vi "CenterFinder_6points.vi"() -> ()   [LabVIEW 2016]
uses:
  Control/ProcessCtl.ctl
  <vilib>/userdefined/High Color/IMAQdx.ctl
  <vilib>/Utility/config.llb/Read Key (String).vi
  <vilib>/Utility/config.llb/Write Key (Double).vi
  <vilib>/vision/driver/NI_Vision_Acquisition_Software.lvlib
  <vilib>/vision/NI_Vision_Development_Module.lvlib
  <vilib>/Utility/config.llb/NI_LVConfig.lvlib
panel:
  out "Array":T1(array[cluster])
  in  "MoveTo":bool
  out "Boolean":bool=TRUE
  in  "GoToXY":bool
  out "Tip Center":cluster{"X":dbl, "Y":dbl, "Z":dbl}
  in  "Minimum Edge Strength":dbl=10.0
  out "Camera Center":cluster{"X":dbl, "Y":dbl, "Z":dbl}
  out "1":bool[](array[boolean])
  in  "LR/TB":enum16{"B2T", "L2R", "R2L", "T2B"}(ring)=enum."R2L"
  in  "Delete":bool caption="Retake"
  in  "Retake":bool caption="Delete"
  in  "Next":bool
  in  "Process":bool
  in  "Acquire":bool
  in  "stop":bool
  out "Image":T2(plugin-control)
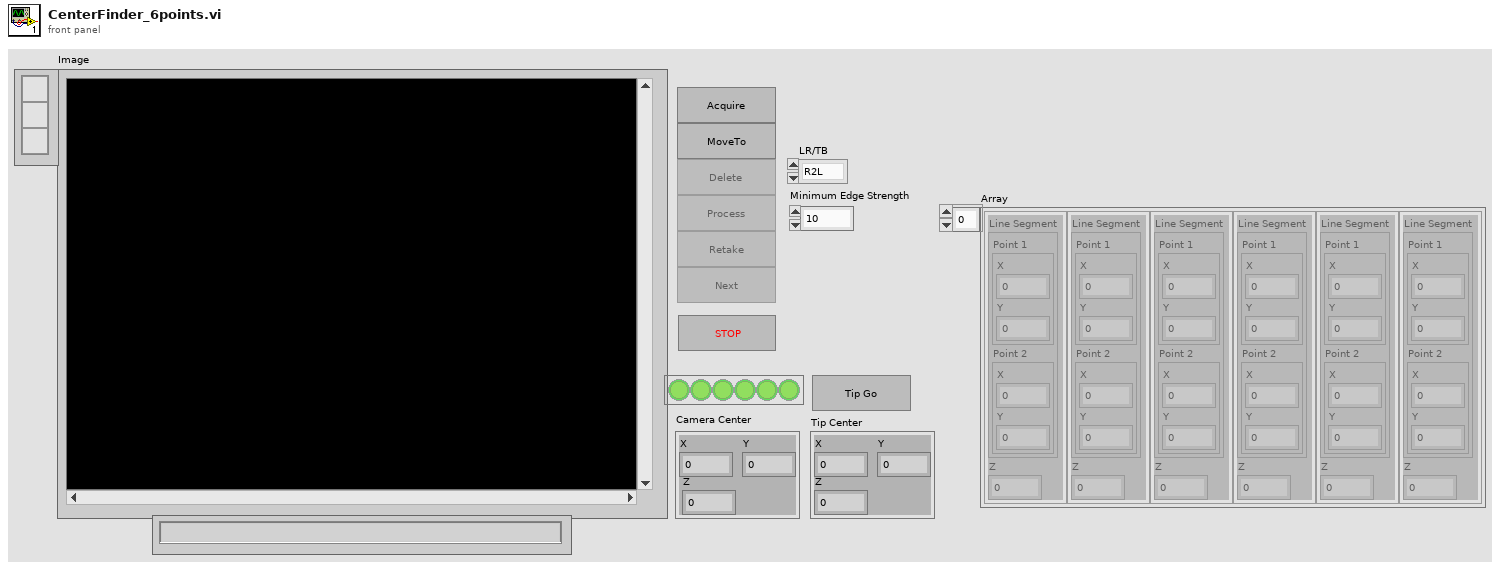
[diagram p1: front panel]
types:
  T1 = cluster{"Line Segment":cluster{"Point 1":cluster{"X":sgl, "Y":sgl}, "Point 2":cluster{"X":sgl, "Y":sgl}}, "Z":dbl}[]
  T2 = typedef "IMAQ Image.ctl" = refnum<image>
  T3 = typedef "IMAQdx.ctl" = refnum<k21>
  T4 = typedef "ProcessCtl.ctl" = enum16{"Idle", "Acquire", "Process", "Abort", "Initialize", "Wait"}
  T5 = typedef "NI_LVConfig.lvlib/Config Data RefNum.ctl" = refnum<k1>
  T6 = enum8{"Enabled", "Disabled", "Disabled and Grayed Out"}
  T7 = cluster{"Line Segment":cluster{"Point 1":cluster{"X":sgl, "Y":sgl}, "Point 2":cluster{"X":sgl, "Y":sgl}}, "Z":dbl}
  T8 = cluster{"Edge Polarity":u16, "Kernel Size":u32, "Width":u32, "Minimum Edge Strength":dbl, "Interpolation Type":u16, "Data Processing Method":u16}
  T9 = typedef "Image Type" = u32
  T10 = typedef "IMAQ Line" = cluster{"Start X":i32, "Start Y":i32, "End X":i32, "End Y":i32}
  T11 = typedef "ROI Descriptor" = cluster{"Global Rectangle":i32[], "Contours":cluster{"ID":enum32{"External", "Internal"}, "Type":u32, "Coordinates":i32[]}[]}
  T12 = typedef "Edge New.ctl" = cluster{"Location (Pixel)":cluster{"X":sgl, "Y":sgl}, "Location (Real-World)":cluster{"X":sgl, "Y":sgl}, "Distance (Pixel)":dbl, "Distance (Real-World)":dbl, "Strength":dbl, "Noise":dbl, "Rising?":bool}
  T13 = cluster{"Point 1":cluster{"X":sgl, "Y":sgl}, "Point 2":cluster{"X":sgl, "Y":sgl}}
  T14 = typedef "ControllerDiagPacket.ctl" = cluster{"Number of Diag Packets":i32, "Axes":T15[], "error":errorcluster}
  T15 = typedef "AxisDiagPacket.ctl" = cluster{"Axis Name":string, "Analog Input 0":dbl, "Analog Input 1":dbl, "Axis Fault (num)":i32, "Axis Fault (str)":string, "Axis Fault (bits)":cluster{"AmplifierFault":bool, "AmplifierTemperatureFault":bool, "CcwEndOfTravelLimitFault":bool, "CcwSoftwareLimitFault":bool, "CommunicationLostFault":bool, "CwEndOfTravelLimitFault":bool, "CwSoftwareLimitFault":bool, "EmergencyStopFault":bool, "EncoderFault":bool, "ExternalFault":bool, "FeedbackScalingFault":bool, "GantryMisalignFault ":bool, "HallSensorFault":bool, "InPositionTimeoutFault":bool, "InternalFault":bool, "MarkerSearchFault":bool, "MaxVelocityCommandFault":bool, "MissedInterruptFault":bool, "MotorTemperatureFault":bool, "None":bool, "OverCurrentFault":bool, "PositionErrorFault":bool, "PositionFeedbackFault":bool, "PowerSupplyFault":bool, "ProbeInputFault":bool, "SafeZoneFault":bool, "VelocityErrorFault":bool, "VelocityFeedbackFault":bool, "VoltageClampFault":bool}, "Axis Status (num)":i32, "Axis Status (str)":string, "Axis Status (bits)":cluster{"BacklashActive":bool, "CalibrationEnabled1D":bool, "CalibrationEnabled2D":bool, "CommandValid":bool, "DriveAbortPending":bool, "DrivePending":bool, "Enabling":bool, "GainMappingEnabled":bool, "GantryAligned":bool, "GantryRealigning":bool, "Homed":bool, "Homing":bool, "IFOVEnabled":bool, "JogGenerating":bool, "Jogging":bool, "JoystickControl":bool, "MasterSlaveControl":bool, "MotionBlocked":bool, "MotionClamped":bool, "MoveDone":bool, "None":bool, "NotVirtual":bool, "Profiling":bool, "Stability0":bool, "Stability1":bool, "TrajectoryFiltering":bool, "WaitDone":bool}, "Current Command":sgl, "Current Error":sgl, "Current Feedback":sgl, "Digital Inputs":i32, "Digital Outputs":i32, "Drive Status":i32, "Drive Status (str)":string, "Drive Status (bits)":cluster{"AccelerationPhase":bool, "AutofocusActive":bool, "BrakeOutput":bool, "CcwEndOfTravelLimitInput":bool, "CosineEncoderError":bool, "CurrentClamp":bool, "CwEndOfTravelLimitInput":bool, "DecelerationPhase":bool, "DualLoopActive":bool, "EmergencyStopInput":bool, "Enabled":bool, "EncoderClipping":bool, "GalvoCalibrationEnabled":bool, "GalvoPowerCorrection":bool, "HallAInput":bool, "HallBInput":bool, "HallCInput":bool, "HighResolutionMode":bool, "HomeLimitInput":bool, "InPosition":bool, "InPosition2":bool, "MarkerInput":bool, "MarkerLatch":bool, "MoveActive":bool, "NoMotorSupply":bool, "None":bool, "PowerLimiting":bool, "ProgrammingFlash":bool, "ProgrammingMXH":bool, "PSOHaltLatch":bool, "ServoControl":bool, "SineEncoderError":bool}, "Position Feedback Auxiliary":dbl, "Position Command":dbl, "Position Error":dbl, "Position Feedback":dbl, "Program Position Command":dbl, "Program Position Error":dbl, "Program Position Feedback":dbl, "Velocity Command":dbl, "Velocity Error":dbl, "Velocity Feedback":dbl}
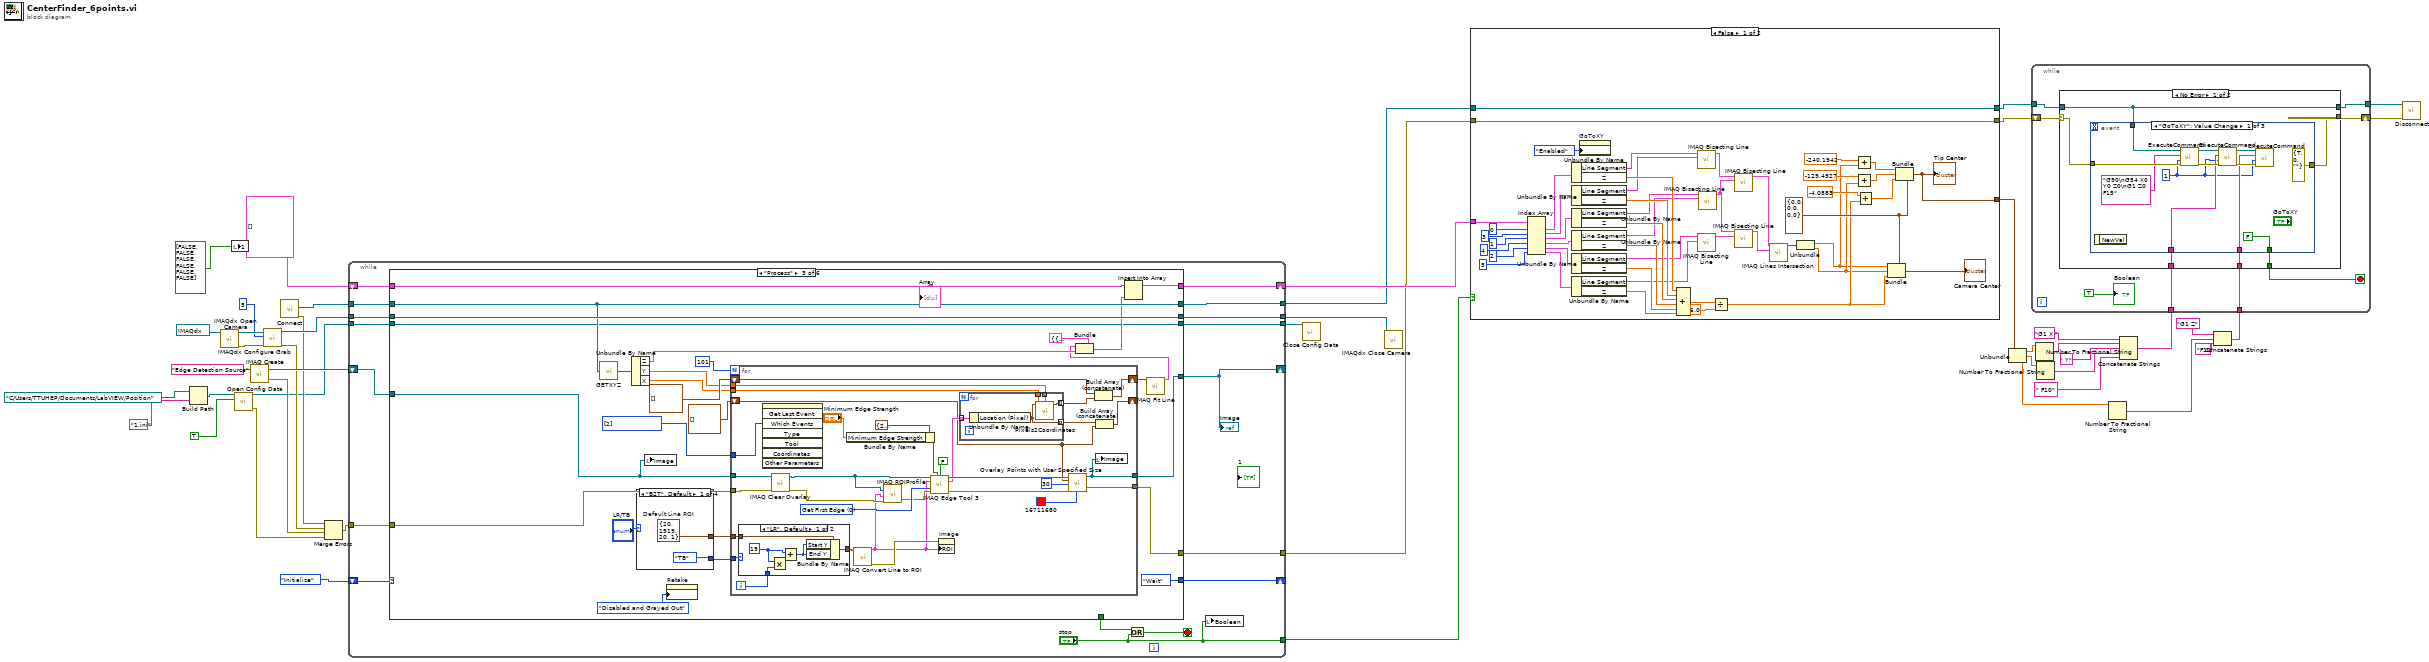
[diagram p0: block diagram]
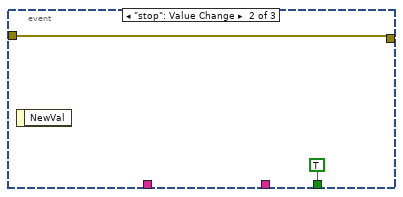
[diagram p2: hidden frame]
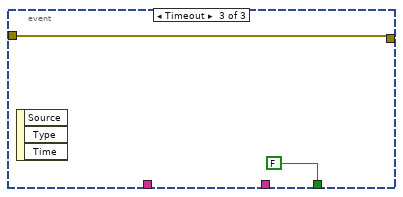
[diagram p3: hidden frame]
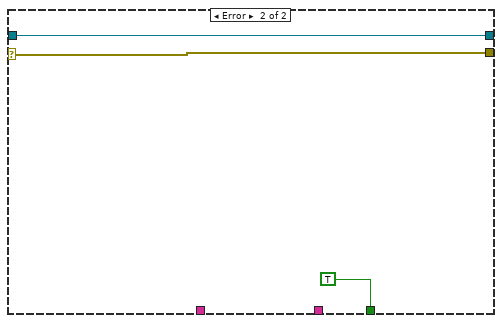
[diagram p4: hidden frame]
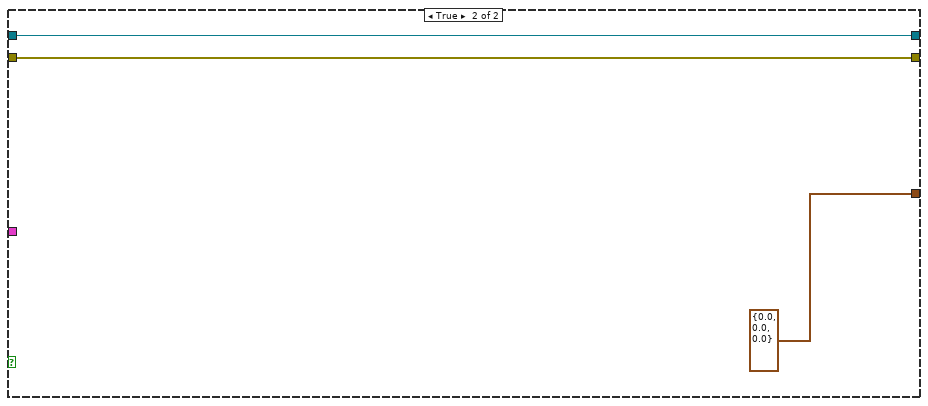
[diagram p5: hidden frame]
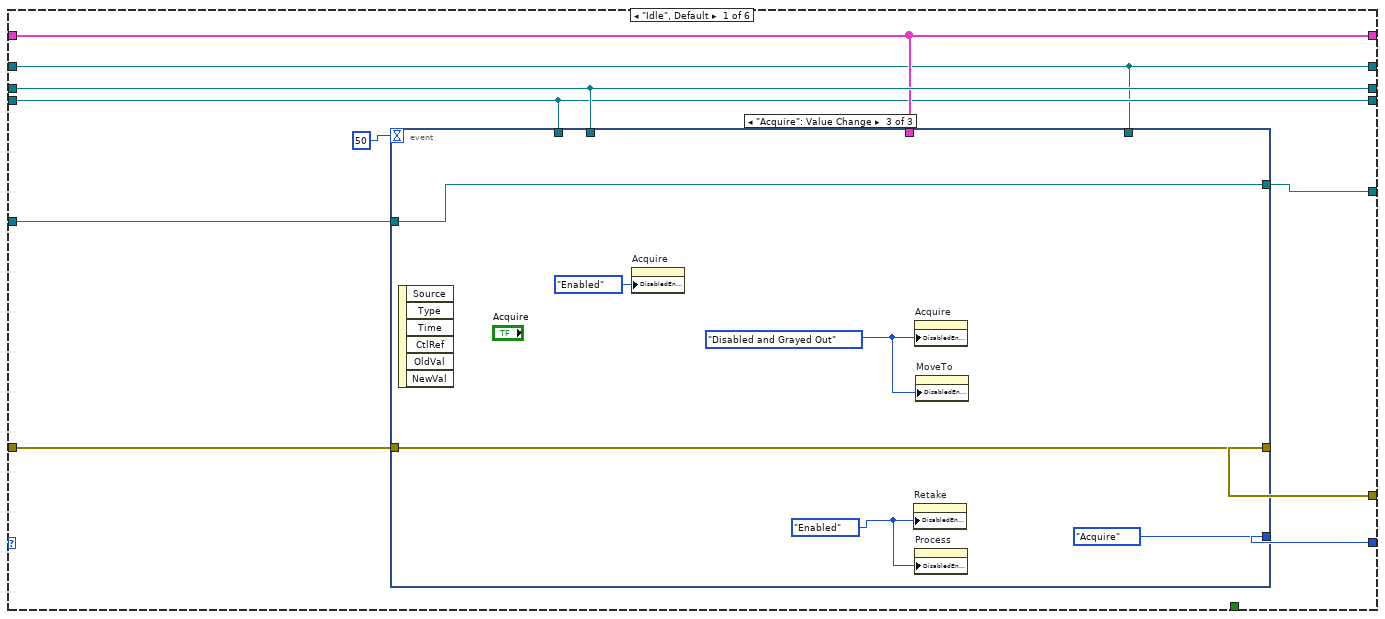
[diagram p6: hidden frame]
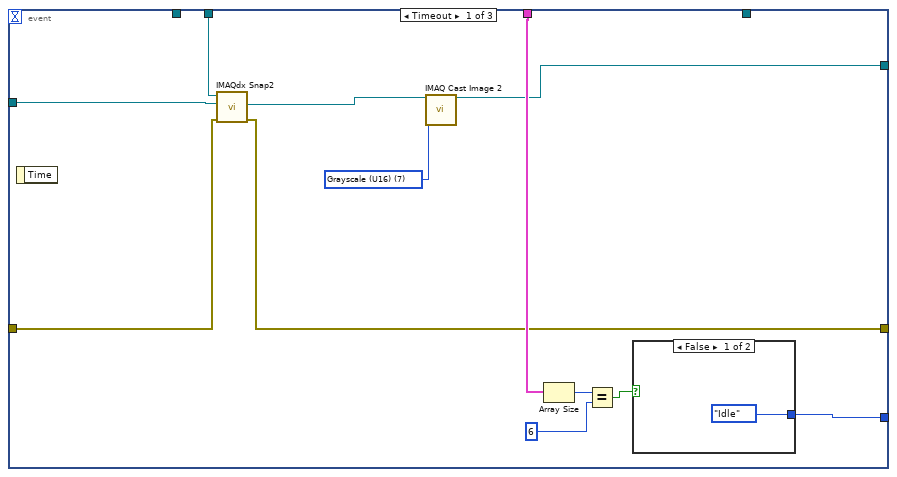
[diagram p7: hidden frame]
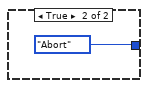
[diagram p8: hidden frame]
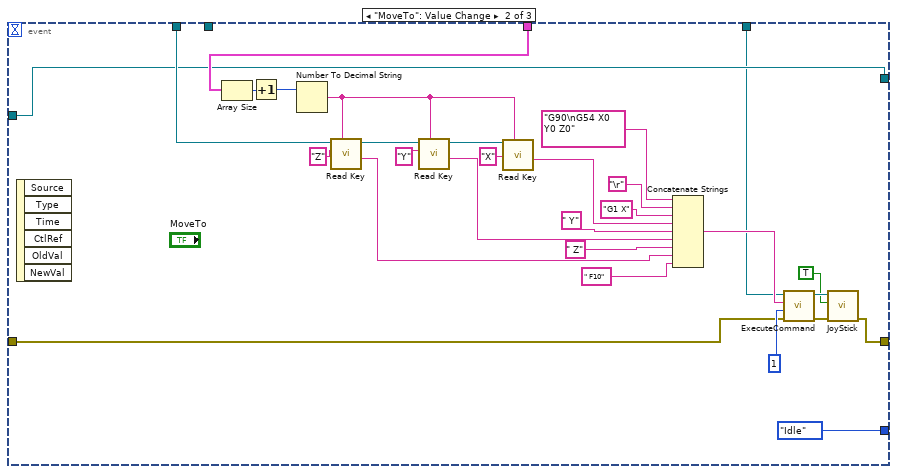
[diagram p9: hidden frame]
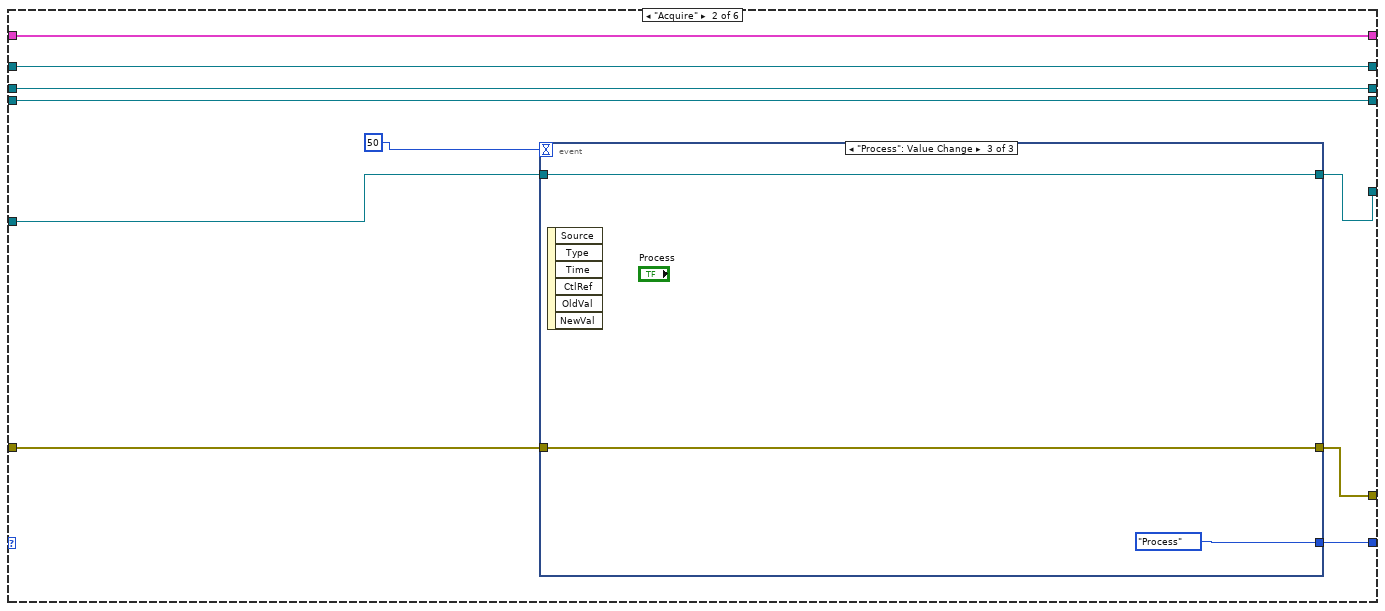
[diagram p10: hidden frame]
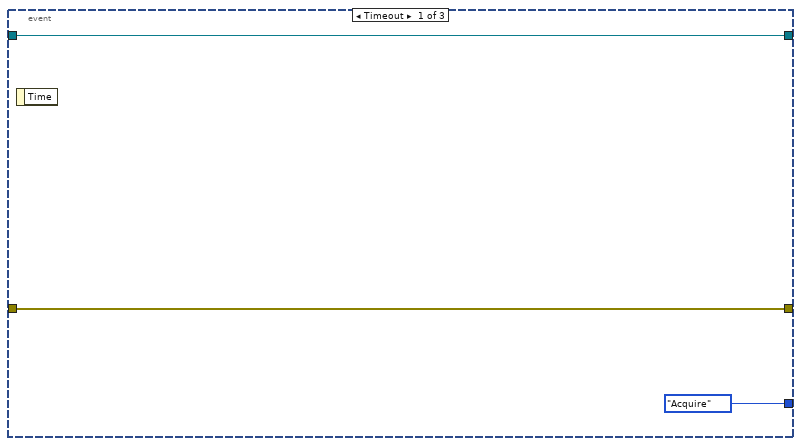
[diagram p11: hidden frame]
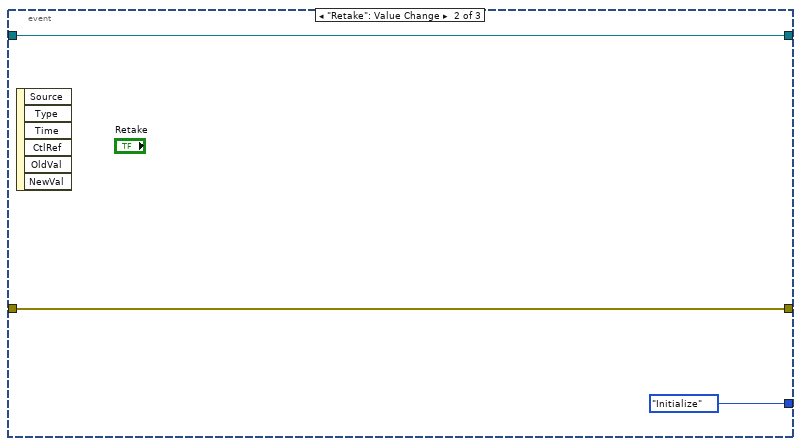
[diagram p12: hidden frame]
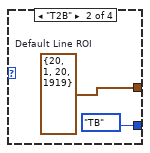
[diagram p13: hidden frame]
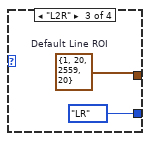
[diagram p14: hidden frame]
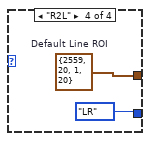
[diagram p15: hidden frame]
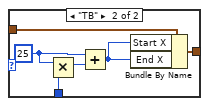
[diagram p16: hidden frame]
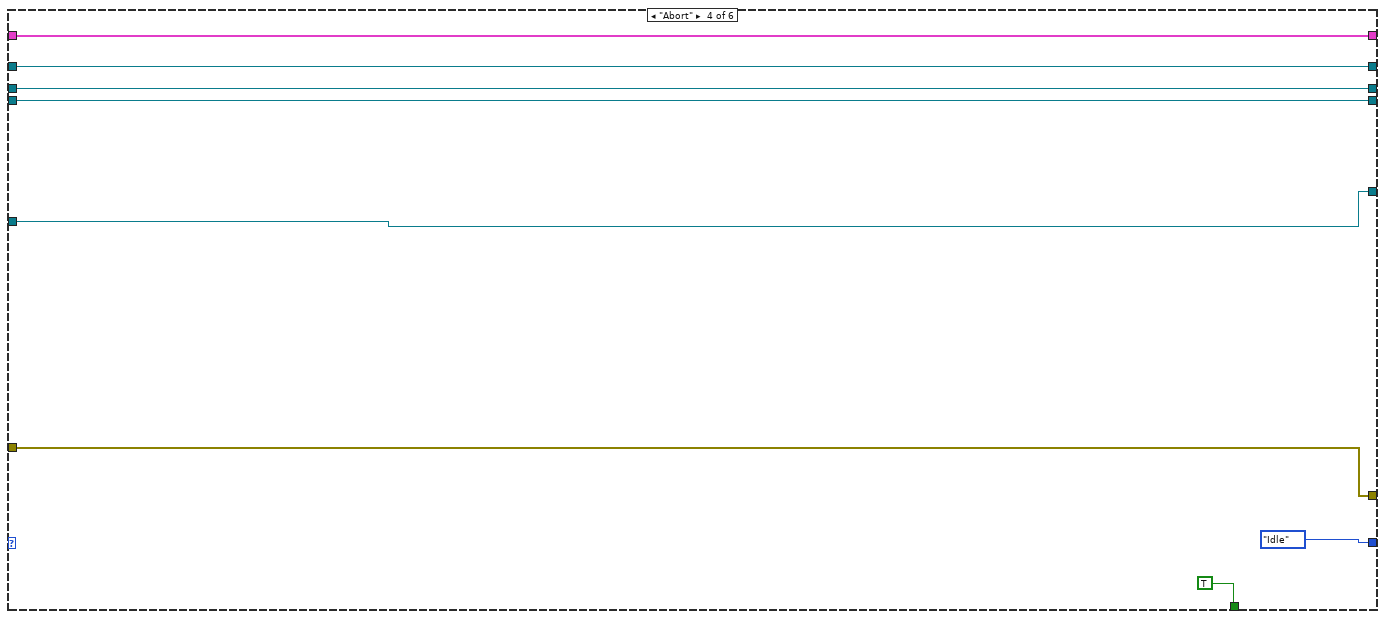
[diagram p17: hidden frame]
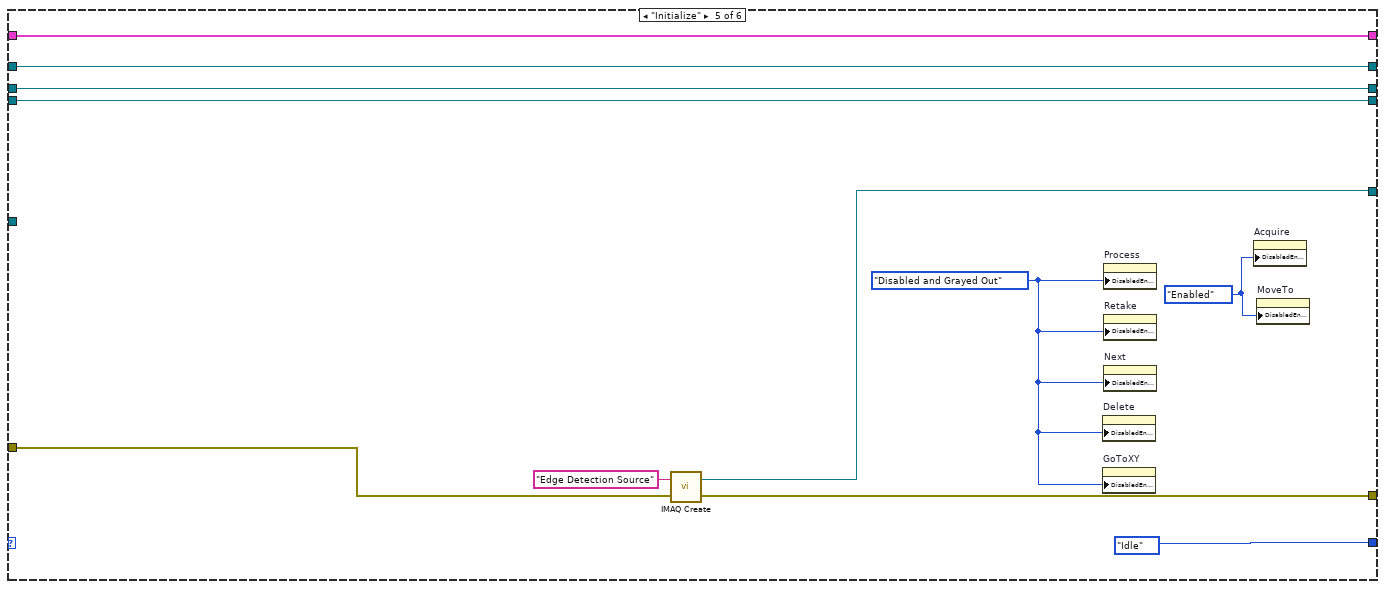
[diagram p18: hidden frame]
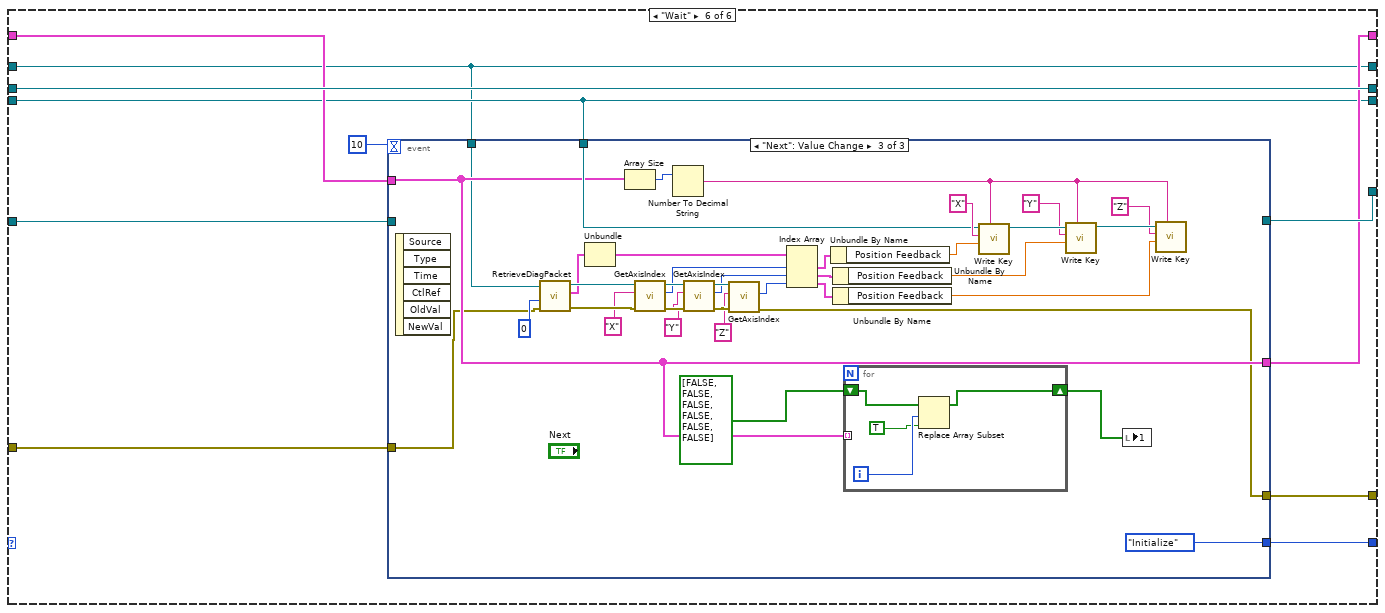
[diagram p19: hidden frame]
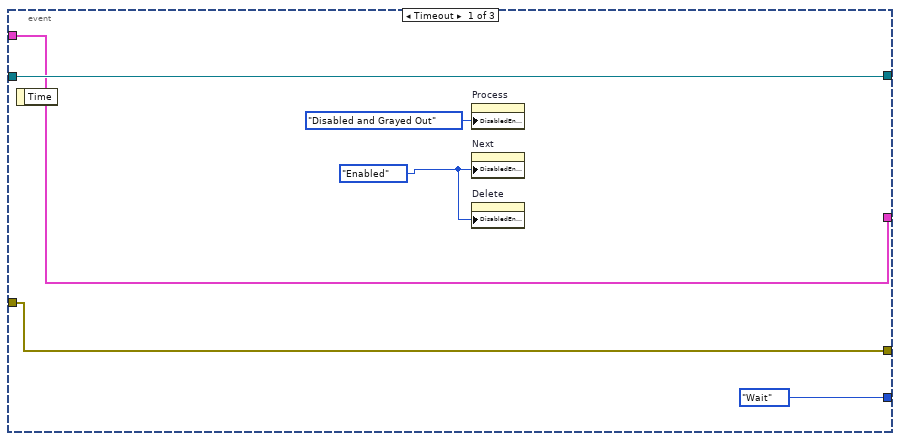
[diagram p20: hidden frame]
diagram:
  n1 = Build Path(base path=path "C:/Users/TTUHEP/Documents/LabVIEW/Position", name or relative path="1.ini") -> (appended path=w6:path)
  n2 = call <vilib>:"IMAQdx Open Camera.vi"("Session In"=T3 "cam0") -> ("error out"=w42:errorcluster, "Session Out"=w43:T3)  [unwired: 9 in]
  n3 = local write "1"(bool[] [FALSE, FALSE, FALSE, FALSE, FALSE, FALSE] ("1 2")) -> ()
  n4 = call <vilib>:"Open Config Data.vi"("create file if necessary (T)"=TRUE, "configuration file path"=w6) -> ("error out"=w5:errorcluster, "refnum"=w4:T5)  [unwired: 7 in, 1 out]
  n5 = call "IMAQ Create"("Image Name"="Edge Detection Source") -> ("New Image"=w40:T2, "error out"=w36:errorcluster)  [unwired: 4 in]
  n6 = call <vilib>:"IMAQdx Configure Grab.vi"("error in"=w42, "Number of Buffers"=u32 5, "Session In"=w43) -> ("error out"=w37:errorcluster, "Session Out"=w44:T3)  [unwired: 7 in]
  n7 = call "Connect.vi"() -> ("error out"=w15:errorcluster, "controller"=w16:refnum<k24>)  [unwired: 10 in]
  n8 = Merge Errors(w15, w37, w36, w5) -> (w35:errorcluster)
  n9 = while {
    tunnel: w44 -> [w53]
    tunnel: [w52] -> w38
    shift-right: [w59] -> _
    shift-left: w40 -> [w57]
    tunnel: w16 -> [w55]
    tunnel: [w54] -> w28
    tunnel: w35 -> [w62]
    shift-right: [w60] -> _
    shift-left: ProcessCtl."Initialize" -> [w61]
    tunnel: [w58] -> w29
    shift-right: [w49] -> w31
    shift-left: T1 [] -> [w56]
    tunnel: ["stop"] -> w30
    tunnel: w4 -> [w47]
    tunnel: [w46] -> w3
    stop <- w50 stop-if-true
    n10 = case shown="\"Process\"" w61 {
      tunnel: w62 -> [w72 w127 w165 w226 w239 w246]
      tunnel: [w69 w128 ProcessCtl."Wait" ProcessCtl."Idle" ProcessCtl."Idle" w251] -> w60
      tunnel: w57 -> [w71 w131 w147 w229 _ w253]
      tunnel: [w70 w130 w157 w229 w240 w252] -> w59
      tunnel: [w68 w126 w151 w226 w238 w247] -> w58
      tunnel: w56 -> [w66 w125 w153 w231 w237 w249]
      tunnel: [w66 w125 w152 w231 w237 w248] -> w49
      tunnel: w55 -> [w64 w124 w154 w225 w236 w243]
      tunnel: [w64 w124 w154 w225 w236 w243] -> w54
      tunnel: w53 -> [w67 w123 w155 w230 w235 w250]
      tunnel: [w67 w123 w155 w230 w235 w250] -> w52
      tunnel: [_ _ _ TRUE _ _] -> w51
      tunnel: [w65 w122 w141 w224 w233 w244] -> w46
      tunnel: w47 -> [w65 w122 w141 w224 w233 w244]
      frame "Idle", Default {
        n11 = event shown="[2] \"Acquire\": Value Change" {
          selector: _ -> [_ _ _]
          dyn-events: _ -> [_ _ _]
          timeout: 50 -> [_ _ _]
          tunnel: w72 -> [w75 w88 w118]
          tunnel: w71 -> [w77 w93 w120]
          tunnel: w67 -> [w76 _ _]
          tunnel: [w78 w93 w120] -> w70
          tunnel: [w84 ProcessCtl."Idle" ProcessCtl."Acquire"] -> w69
          tunnel: [w74 w90 w118] -> w68
          tunnel: w66 -> [w83 w114 _]
          tunnel: w65 -> [_ w115 _]
          tunnel: w64 -> [_ w87 _]
          event Timeout {
            w79 = T9 7 items=["Grayscale (U8)", "Grayscale (I16)", "Grayscale (SGL)", "Complex (CSG)", "RGB (U32)", "HSL (U32)", "RGB (U64)", "Grayscale (U16)"] ("Image Type")
            n12 = event-data() -> ()  [unwired: 1 in, 1 out]
            n13 = call <vilib>:"IMAQdx Snap2.vi"("error in"=w75, "Image In"=w77, "Session In"=w76) -> ("error out"=w74:errorcluster, "Image Out"=w73:T2)  [unwired: 6 in, 1 out]
            n14 = call "IMAQ Cast Image 2"("Image Src"=w73, "Image Type"=w79) -> ("Image Dst Out"=w78:T2)  [unwired: 12 in, 1 out]
            n15 = Array Size(array=w83) -> (size(s)=w82:i32)
            n16 = Equal?(x=w82, y=6) -> (x = y?=w80:bool)
            n17 = case shown="False" w80 {
              tunnel: [ProcessCtl."Idle" ProcessCtl."Abort"] -> w84
              frame False {
              }
              frame True {
              }
            }
          }
          event "MoveTo": Value Change {
            n18 = event-data() -> ()  [unwired: 1 in, 6 out]
            n19 = Array Size(array=w114) -> (size(s)=w113:i32)
            n20 = Increment(x=w113) -> (x+1=w95:i32)
            n21 = Number To Decimal String(number=w95) -> (decimal integer string=w112:string)  [unwired: 1 in]
            n22 = call-poly <vilib>:"Read Key.vi"("section"=w112, "key"="Z", "refnum"=w115) -> ("value"=w101:string, "refnum out"=w108:T5)  [unwired: 5 in, 2 out]
            n23 = call-poly <vilib>:"Read Key.vi"("section"=w112, "key"="Y", "refnum"=w108) -> ("value"=w102:string, "refnum out"=w107:T5)  [unwired: 5 in, 2 out]
            n24 = call-poly <vilib>:"Read Key.vi"("section"=w112, "key"="X", "refnum"=w107) -> ("value"=w103:string)  [unwired: 5 in, 3 out]
            n25 = Concatenate Strings("G90\nG54 X0 Y0 Z0", "\r", "G1 X", w103, " Y", w102, " Z", w101, " F10") -> (w97:string)
            n26 = call "ExecuteCommand.vi"("error in (no error)"=w88, "taskId"=1, "Command Code"=w97, "controller in"=w87) -> ("error out"=w91:errorcluster, "controller out"=w92:refnum<k24>)  [unwired: 5 in, 1 out]
            n27 = call "JoyStick.vi"("error in (no error)"=w91, "On/Off"=TRUE, ".NET Refnum in"=w92) -> ("error out"=w90:errorcluster)  [unwired: 7 in, 1 out]
          }
          event "Acquire": Value Change {
            w119 = T6."Enabled" ("Disabled")
            w117 = T6."Disabled and Grayed Out" ("Disabled")
            n28 = event-data() -> ()  [unwired: 1 in, 6 out]
            n29 = property on="Acquire" class="Bool"("DisabledEnum"=T6."Enabled" ("Disabled")) -> ()  [unwired: 2 in, 2 out]
            n30 = property on="Retake" class="Bool"("DisabledEnum"=w119) -> ()  [unwired: 2 in, 2 out]
            n31 = property on="Acquire" class="Bool"("DisabledEnum"=w117) -> ()  [unwired: 2 in, 2 out]
            n32 = property on="Process" class="Bool"("DisabledEnum"=w119) -> ()  [unwired: 2 in, 2 out]
            n33 = property on="MoveTo" class="Bool"("DisabledEnum"=w117) -> ()  [unwired: 2 in, 2 out]
          }
        }
      }
      frame "Acquire" {
        n34 = event shown="[2] \"Process\": Value Change" {
          selector: _ -> [_ _ _]
          dyn-events: _ -> [_ _ _]
          timeout: 50 -> [_ _ _]
          tunnel: w131 -> [w134 w135 w138]
          tunnel: [w134 w135 w138] -> w130
          tunnel: [ProcessCtl."Acquire" ProcessCtl."Initialize" ProcessCtl."Process"] -> w128
          tunnel: w127 -> [w132 w136 w139]
          tunnel: [w132 w136 w139] -> w126
          event Timeout {
            n35 = event-data() -> ()  [unwired: 1 in, 1 out]
          }
          event "Retake": Value Change {
            n36 = event-data() -> ()  [unwired: 1 in, 6 out]
          }
          event "Process": Value Change {
            n37 = event-data() -> ()  [unwired: 1 in, 6 out]
          }
        }
      }
      frame "Process" {
        w166 = i32[] [2] items=["No  event", "Click event", "Draw event", "Move event", "Size event", "Scroll event", "Activate event", "Close event", "Double click event"] ("Events list (all)")
        n38 = call "GETXYZ.vi"(".NET Refnum in"=w154) -> ("XYZ"=w160:cluster{"X":dbl, "Y":dbl, "Z":dbl})
        n39 = Unbundle By Name(w160) -> ("Z"=w144:dbl, "Y"=w159:dbl, "X"=w158:dbl)
        n40 = case shown="\"B2T\", Default" "LR/TB" {
          tunnel: [w168 w170 w171 w173] -> w163
          tunnel: [enum16{"LR", "TB"}."TB" enum16{"LR", "TB"}."TB" enum16{"LR", "TB"}."LR" enum16{"LR", "TB"}."LR"] -> w148
          frame "B2T", Default {
            w168 = T10 {"Start X"=20, "Start Y"=1919, "End X"=20, "End Y"=1}  # Default Line ROI
          }
          frame "T2B" {
            w170 = T10 {"Start X"=20, "Start Y"=1, "End X"=20, "End Y"=1919}  # Default Line ROI
          }
          frame "L2R" {
            w171 = T10 {"Start X"=1, "Start Y"=20, "End X"=2559, "End Y"=20}  # Default Line ROI
          }
          frame "R2L" {
            w173 = T10 {"Start X"=2559, "Start Y"=20, "End X"=1, "End Y"=20}  # Default Line ROI
          }
        }
        n41 = local write "Image"(w147) -> ()
        n42 = property on="Retake" class="Bool"("DisabledEnum"=T6."Disabled and Grayed Out" ("Disabled")) -> ()  [unwired: 2 in, 2 out]
        n43 = for {
          N: 101 -> [_]
          tunnel: w147 -> [w186]
          tunnel: w165 -> [w204]
          shift-right: [w196] -> w161
          shift-left: cluster{"X":sgl, "Y":sgl}[] [] -> [w198]
          tunnel: w166 -> [w190]
          tunnel: [w181] -> w157
          tunnel: [w195] -> w151
          tunnel: w163 -> [w193]
          tunnel: w159 -> [w192]
          tunnel: w158 -> [w191]
          tunnel: w148 -> [w188]
          shift-right: [w180] -> _
          shift-left: cluster{"X":sgl, "Y":sgl}[] [] -> [w178]
          i -> [w206]
          w203 = u16 0 items=["Get First Edge", "Get First + Last Edge", "Get All Edges", "Get Best Edge"] ("Process")
          n44 = case shown="\"LR\", Default" w188 {
            tunnel: w206 -> [w210 w218]
            tunnel: [w212 w214] -> w205
            tunnel: w193 -> [w211 w213]
            frame "LR", Default {
              w207 = 19
              n45 = Multiply(x=w207, y=w210) -> (x*y=w208:i32)
              n46 = Add(x=w207, y=w208) -> (x+y=w209:i32)
              n47 = Bundle By Name(cluster=w211, "Start Y"=w209, "End Y"=w209) -> (w212:T10)
            }
            frame "TB" {
              w216 = 25
              n48 = Multiply(x=w216, y=w218) -> (x*y=w217:i32)
              n49 = Add(x=w216, y=w217) -> (x+y=w215:i32)
              n50 = Bundle By Name(cluster=w213, "Start X"=w215, "End X"=w215) -> (w214:T10)
            }
          }
          n51 = invoke on="Image" class="ImageControl" method="Get Last Event"("Which Events"=w190) -> ()  [unwired: 7 in, 8 out]
          n52 = call "IMAQ Clear Overlay"("error in (no error)"=w204, "Image"=w186) -> ("error out"=w184:errorcluster, "Image Out"=w182:T2)  [unwired: 8 in]
          n53 = Bundle By Name(cluster=T8 {"Edge Polarity"=2, "Kernel Size"=37, "Width"=5, "Minimum Edge Strength"=10.0, "Interpolation Type"=0, "Data Processing Method"=1} ("Edge Options"), "Minimum Edge Strength"="Minimum Edge Strength") -> (w176:T8)
          n54 = call "IMAQ Convert Line to ROI"("Line"=w205) -> ("error out"=w189:errorcluster, "ROI Descriptor"=w183:T11)  [unwired: 8 in]
          n55 = call "IMAQ ROIProfile"("error in (no error)"=w184, "ROI Descriptor"=w183, "Image"=w182) -> ("error out"=w185:errorcluster)  [unwired: 1 in, 4 out]
          n56 = call "IMAQ Edge Tool 3"("Image"=w182, "Edge Options"=w176, "Optimized Mode"=FALSE, "ROI Descriptor"=w183, "Process"=w203, "error in (no error)"=w185) -> ("Image (duplicate)"=w201:T2, "Edge Information"=w187:T12[], "error out"=w200:errorcluster)  [unwired: 5 in, 2 out]
          n57 = property on="Image" class="ImageControl"(error in=w189, "ROI"=w183) -> ()  [unwired: 1 in, 2 out]
          n58 = for {
            tunnel: w187 -> [w223] mode=indexing
            tunnel: [w222] -> w197 mode=indexing
            tunnel: w192 -> [w221]
            tunnel: w191 -> [w220]
            tunnel: [w219] -> w179 mode=indexing
            n59 = Unbundle By Name(w223) -> ("Location (Pixel)"=w219:cluster{"X":sgl, "Y":sgl})
            n60 = call "Pixels2Coordinates.vi"("Y"=w221, "X"=w220, "Location (Pixel)"=w219) -> ("output cluster"=w222:cluster{"X":sgl, "Y":sgl})  [unwired: 8 in]
          }
          n61 = call "Overlay Points with User Specified Size.vi"("Color"=u32 16711680, "error in"=w200, "Point Diameter (5)"=30, "Points"=w178, "Image In"=w201) -> ("error out"=w195:errorcluster, "Image Out"=w181:T2)  [unwired: 5 in]
          n62 = Build Array (concatenate)(w198, w197) -> (w196:cluster{"X":sgl, "Y":sgl}[])
          n63 = Build Array (concatenate)(w179, w178) -> (w180:cluster{"X":sgl, "Y":sgl}[])
          n64 = local write "Image"(w181) -> ()
        }
        n65 = call "IMAQ Fit Line"("Points"=w161) -> ("Line Segment"=w143:T13)  [unwired: 5 in, 5 out]
        n66 = Bundle(cluster=T7 {"Line Segment"={"Point 1"={"X"=0.0, "Y"=0.0}, "Point 2"={"X"=0.0, "Y"=0.0}}, "Z"=0.0}, "Line Segment"=w143, "Z"=w144) -> (w142:T7)
        n67 = Insert Into Array(array=w153, new element=w142) -> (w152:T1)  [unwired: 1 in]
        "Array" <- w153
      }
      frame "Abort" {
      }
      frame "Initialize" {
        w234 = T6."Disabled and Grayed Out" ("Disabled")
        w232 = T6."Enabled" ("Disabled")
        n68 = call "IMAQ Create"("Image Name"="Edge Detection Source", "error in (no error)"=w239) -> ("New Image"=w240:T2, "error out"=w238:errorcluster)  [unwired: 3 in]
        n69 = property on="Delete" class="Bool"("DisabledEnum"=w234) -> ()  [unwired: 2 in, 2 out]
        n70 = property on="GoToXY" class="Bool"("DisabledEnum"=w234) -> ()  [unwired: 2 in, 2 out]
        n71 = property on="Process" class="Bool"("DisabledEnum"=w234) -> ()  [unwired: 2 in, 2 out]
        n72 = property on="Retake" class="Bool"("DisabledEnum"=w234) -> ()  [unwired: 2 in, 2 out]
        n73 = property on="Next" class="Bool"("DisabledEnum"=w234) -> ()  [unwired: 2 in, 2 out]
        n74 = property on="Acquire" class="Bool"("DisabledEnum"=w232) -> ()  [unwired: 2 in, 2 out]
        n75 = property on="MoveTo" class="Bool"("DisabledEnum"=w232) -> ()  [unwired: 2 in, 2 out]
      }
      frame "Wait" {
        n76 = event shown="[2] \"Next\": Value Change" {
          selector: _ -> [_ _ _]
          dyn-events: _ -> [_ _ _]
          timeout: 10 -> [_ _ _]
          tunnel: w253 -> [w259 w262 _]
          tunnel: [w259 w262 _] -> w252
          tunnel: [ProcessCtl."Wait" ProcessCtl."Initialize" ProcessCtl."Initialize"] -> w251
          tunnel: w249 -> [w257 w265 w290]
          tunnel: [w257 w264 w290] -> w248
          tunnel: [w256 w260 w280] -> w247
          tunnel: w246 -> [w256 w260 w266]
          tunnel: w244 -> [_ _ w291]
          tunnel: w243 -> [_ _ w267]
          event Timeout {
            w254 = T6."Enabled" ("Disabled")
            n77 = event-data() -> ()  [unwired: 1 in, 1 out]
            n78 = property on="Process" class="Bool"("DisabledEnum"=T6."Disabled and Grayed Out" ("Disabled")) -> ()  [unwired: 2 in, 2 out]
            n79 = property on="Next" class="Bool"("DisabledEnum"=w254) -> ()  [unwired: 2 in, 2 out]
            n80 = property on="Delete" class="Bool"("DisabledEnum"=w254) -> ()  [unwired: 2 in, 2 out]
          }
          event "Delete": Value Change {
            n81 = event-data() -> ()  [unwired: 1 in, 6 out]
            n82 = Delete From Array(array=w265, index=0) -> (array with subset deleted=w264:T1)  [unwired: 1 in, 1 out]
          }
          event "Next": Value Change {
            n83 = event-data() -> ()  [unwired: 1 in, 6 out]
            n84 = call "RetrieveDiagPacket.vi"("error in (no error)"=w266, "axisMask"=0, "Controller In"=w267) -> ("error out"=w283:errorcluster, "ControllerDiagPacket"=w286:T14, "Controller Out"=w289:refnum<k24>)  [unwired: 6 in]
            n85 = Unbundle(w286) -> ("Axes"=w285:T15[])  [unwired: 2 out]
            n86 = Array Size(array=w290) -> (size(s)=w298:i32)
            n87 = call "GetAxisIndex.vi"("error in (no error)"=w283, "axis name"="X", "controller in"=w289) -> ("error out"=w282:errorcluster, "axis index"=w277:i32, "controller out"=w288:refnum<k24>)  [unwired: 6 in]
            n88 = Number To Decimal String(number=w298) -> (decimal integer string=w297:string)  [unwired: 1 in]
            n89 = call "GetAxisIndex.vi"("error in (no error)"=w282, "axis name"="Y", "controller in"=w288) -> ("error out"=w281:errorcluster, "axis index"=w278:i32, "controller out"=w287:refnum<k24>)  [unwired: 6 in]
            n90 = call "GetAxisIndex.vi"("error in (no error)"=w281, "axis name"="Z", "controller in"=w287) -> ("error out"=w280:errorcluster, "axis index"=w279:i32)  [unwired: 6 in, 1 out]
            n91 = Index Array(array=w285, index #1=w277, index #2=w278, index #3=w279) -> (element #1=w276:T15, element #2=w275:T15, element #3=w274:T15)
            n92 = Unbundle By Name(w276) -> ("Position Feedback"=w273:dbl)
            n93 = Unbundle By Name(w275) -> ("Position Feedback"=w272:dbl)
            n94 = Unbundle By Name(w274) -> ("Position Feedback"=w271:dbl)
            n95 = for {
              tunnel: w290 -> [_] mode=indexing
              shift-right: [w302] -> w299
              shift-left: bool[] [FALSE, FALSE, FALSE, FALSE, FALSE, FALSE] ("1 2") -> [w305]
              i -> [w304]
              n96 = Replace Array Subset(array=w305, new element=TRUE, index=w304) -> (w302:bool[])
            }
            n97 = call-poly <vilib>:"Write Key.vi"("section"=w297, "value"=w273, "key"="X", "refnum"=w291) -> ("refnum out"=w296:T5)  [unwired: 5 in, 2 out]
            n98 = call-poly <vilib>:"Write Key.vi"("section"=w297, "value"=w272, "key"="Y", "refnum"=w296) -> ("refnum out"=w295:T5)  [unwired: 5 in, 2 out]
            n99 = local write "1"(w299) -> ()
            n100 = call-poly <vilib>:"Write Key.vi"("section"=w297, "value"=w271, "key"="Z", "refnum"=w295) -> ()  [unwired: 5 in, 3 out]
          }
        }
      }
    }
    "Image" <- w59
    n101 = Or(x=w51, y="stop") -> (x .or. y?=w50:bool)
    n102 = local write "Boolean"("stop") -> ()
  }
  n103 = call <vilib>:"Close Config Data.vi"("refnum"=w3) -> ()  [unwired: 9 in, 2 out]
  n104 = call <vilib>:"IMAQdx Close Camera.vi"("Session In"=w38) -> ()  [unwired: 10 in, 1 out]
  n105 = case shown="False" w30 {
    tunnel: w31 -> [w353 _]
    tunnel: w29 -> [w320 w355]
    tunnel: w28 -> [w306 w356]
    tunnel: [w306 w356] -> w26
    tunnel: [w320 w355] -> w27
    tunnel: [w311 cluster{"X":dbl, "Y":dbl, "Z":dbl} {"X"=0.0, "Y"=0.0, "Z"=0.0}] -> w25
    frame False {
      w318 = cluster{"X":dbl, "Y":dbl, "Z":dbl} {"X"=0.0, "Y"=0.0, "Z"=0.0}
      n106 = Index Array(array=w353, index #1=0, index #2=3, index #3=1, index #4=4, index #5=2, index #6=5) -> (element #1=w349:T7, element #2=w348:T7, element #3=w347:T7, element #4=w340:T7, element #5=w339:T7, element #6=w321:T7)
      n107 = Unbundle By Name(w349) -> ("Line Segment"=w332:T13, "Z"=w338:dbl)
      n108 = Unbundle By Name(w348) -> ("Line Segment"=w331:T13, "Z"=w337:dbl)
      n109 = Unbundle By Name(w347) -> ("Line Segment"=w330:T13, "Z"=w336:dbl)
      n110 = Unbundle By Name(w340) -> ("Line Segment"=w329:T13, "Z"=w335:dbl)
      n111 = Unbundle By Name(w339) -> ("Line Segment"=w328:T13, "Z"=w334:dbl)
      n112 = Unbundle By Name(w321) -> ("Line Segment"=w327:T13, "Z"=w333:dbl)
      n113 = property on="GoToXY" class="Bool"("DisabledEnum"=T6."Enabled" ("Disabled")) -> ()  [unwired: 2 in, 2 out]
      n114 = Compound Arithmetic op=ADD(w338, w337, w336, w335, w334, w333) -> (w346:dbl)
      n115 = call "IMAQ Bisecting Line"("Line 2"=w331, "Line 1"=w332) -> ("Bisecting Line"=w326:T13)  [unwired: 8 in, 1 out]
      n116 = call "IMAQ Bisecting Line"("Line 2"=w327, "Line 1"=w328) -> ("Bisecting Line"=w324:T13)  [unwired: 8 in, 1 out]
      n117 = call "IMAQ Bisecting Line"("Line 2"=w329, "Line 1"=w330) -> ("Bisecting Line"=w325:T13)  [unwired: 8 in, 1 out]
      n118 = Divide(x=w346, y=6.0) -> (x/y=w310:dbl)
      n119 = call "IMAQ Bisecting Line"("Line 2"=w325, "Line 1"=w326) -> ("Bisecting Line"=w323:T13)  [unwired: 8 in, 1 out]
      n120 = call "IMAQ Bisecting Line"("Line 2"=w324, "Line 1"=w325) -> ("Bisecting Line"=w322:T13)  [unwired: 8 in, 1 out]
      n121 = call "IMAQ Lines Intersection"("Line 2"=w322, "Line 1"=w323) -> ("Intersection Point"=w344:cluster{"X":sgl, "Y":sgl})  [unwired: 7 in, 2 out]
      n122 = Unbundle(w344) -> ("X"=w308:sgl, "Y"=w309:sgl)
      n123 = Add(x=-240.1942, y=w308) -> (x+y=w314:dbl)
      n124 = Add(x=-129.4927, y=w309) -> (x+y=w313:dbl)
      n125 = Add(x=-4.0883, y=w310) -> (x+y=w312:dbl)
      n126 = Bundle(cluster=w318, "X"=w308, "Y"=w309, "Z"=w310) -> (→"Camera Center":cluster{"X":dbl, "Y":dbl, "Z":dbl})
      n127 = Bundle(cluster=w318, "X"=w314, "Y"=w313, "Z"=w312) -> (w311:cluster{"X":dbl, "Y":dbl, "Z":dbl})
      "Tip Center" <- w311
    }
    frame True {
    }
  }
  n128 = Unbundle(w25) -> ("X"=w24:dbl, "Y"=w23:dbl, "Z"=w13:dbl)
  n129 = Number To Fractional String(number=w24) -> (F-format string=w21:string)  [unwired: 3 in]
  n130 = Number To Fractional String(number=w23) -> (F-format string=w19:string)  [unwired: 3 in]
  n131 = Number To Fractional String(number=w13) -> (F-format string=w12:string)  [unwired: 3 in]
  n132 = Concatenate Strings("G1 X ", w21, " Y", w19, " F10") -> (w17:string)
  n133 = Concatenate Strings("G1 Z", w12, "F10") -> (w10:string)
  n134 = while {
    shift-right: [w361] -> w1
    shift-left: w27 -> [w364]
    tunnel: w17 -> [w359]
    tunnel: w26 -> [w363]
    tunnel: [w362] -> w2
    tunnel: w10 -> [w357]
    stop <- w360 stop-if-true
    n135 = case shown="No Error" w364 {
      selector: w364 -> [w370 w388]
      tunnel: w363 -> [w369 w389]
      tunnel: [w369 w389] -> w362
      tunnel: [w367 w388] -> w361
      tunnel: [w368 TRUE] -> w360
      tunnel: w359 -> [w366 _]
      tunnel: w357 -> [w365 _]
      frame No Error {
        n136 = event shown="[0] \"GoToXY\": Value Change" {
          selector: _ -> [_ _ _]
          dyn-events: _ -> [_ _ _]
          timeout: _ -> [_ _ _]
          tunnel: w370 -> [w382 w383 w386]
          tunnel: w369 -> [w380 _ _]
          tunnel: [FALSE TRUE FALSE] -> w368
          tunnel: [errorcluster {"status"=TRUE, "code"=0, "source"=""} ("error IO") w383 w386] -> w367
          tunnel: w366 -> [w376 _ _]
          tunnel: w365 -> [w372 _ _]
          event "GoToXY": Value Change {
            w371 = 1
            n137 = event-data() -> ()  [unwired: 1 in, 1 out]
            n138 = call "ExecuteCommand.vi"("error in (no error)"=w382, "taskId"=w371, "Command Code"="G90\nG54 X0 Y0 Z0\nG1 Z0 F15", "controller in"=w380) -> ("error out"=w377:errorcluster, "controller out"=w381:refnum<k24>)  [unwired: 5 in, 1 out]
            n139 = call "ExecuteCommand.vi"("error in (no error)"=w377, "taskId"=w371, "Command Code"=w376, "controller in"=w381) -> ("error out"=w373:errorcluster, "controller out"=w374:refnum<k24>)  [unwired: 5 in, 1 out]
            n140 = call "ExecuteCommand.vi"("error in (no error)"=w373, "taskId"=w371, "Command Code"=w372, "controller in"=w374) -> ()  [unwired: 5 in, 3 out]
          }
          event "stop": Value Change {
            n141 = event-data() -> ()  [unwired: 1 in, 1 out]
          }
          event Timeout {
            n142 = event-data() -> ()  [unwired: 1 in, 3 out]
          }
        }
      }
      frame Error {
      }
    }
    "Boolean" <- TRUE
  }
  n143 = call "Disconnect.vi"("error in (no error)"=w1, "controller"=w2) -> ()  [unwired: 9 in, 1 out]
